vi "Determine Setpoint.vi"(8 "error in (no error)":errorcluster, 10 "Elevator State":T1) -> (0 "error out":errorcluster, 2 "Setpoint":dbl)   [LabVIEW 2014]
doc: "Determines the setpoint for Elevator PID.vi as either a manual setpoint or a preset one"
uses:
  Elevator States.ctl
  Elevator Setpoints.ctl
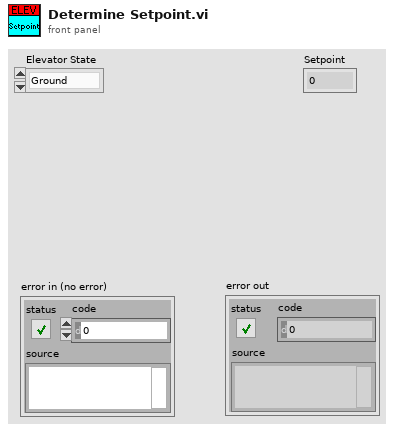
[diagram p1: front panel]
types:
  T1 = typedef "Elevator States.ctl" = enum16{"Ground", "Tote 1", "Tote 2", "Tote 3", "Tote 4", "Tote 5", "Tote 6"}
  T2 = typedef "Elevator Setpoints.ctl" = dbl[]
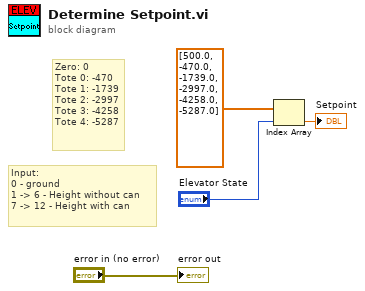
[diagram p0: block diagram]
diagram:
  # "Zero: 0\nTote 0: -470\nTote 1: -1739\nTote 2: -2997\nTote 3: -4258\nTote 4: -5287"
  # "Input:\n0 - ground\n1 -> 6 - Height without can\n7 -> 12 - Height with can"
  n1 = Index Array(array=T2 [500.0, -470.0, -1739.0, -2997.0, -4258.0, -5287.0] ("State Heights"), index="Elevator State") -> (element=→"Setpoint":dbl)
  "error out" <- "error in (no error)"
